vi "Servo MSMT Set Servo Type in Measurement Name.vi"(8 "error in (no error)":errorcluster, 11 "Servo to Power Out in":refnum<class "Servo to Power Out.lvclass">) -> (0 "error out":errorcluster, 3 "Servo to Power Out out":refnum<class "Servo to Power Out.lvclass">)   [LabVIEW 2018, in "Servo to Power Out.lvlib" / "Servo to Power Out.lvclass"]
uses:
  Servo to Power Out.lvclass
  C:/Sequence Automation/Plugins/Measurement Interface.lvlibp/Measurement Interface.lvclass
  Plugins/Measurement Interface.lvlibp/Private Methods/Measurement Name/Read Measurement Name.vi
  Plugins/Measurement Interface.lvlibp/Private Methods/Measurement Name/Write Measurement Name.vi
  Plugins/Measurements/Servo MSMT.lvlibp/Servo MSMT.lvclass
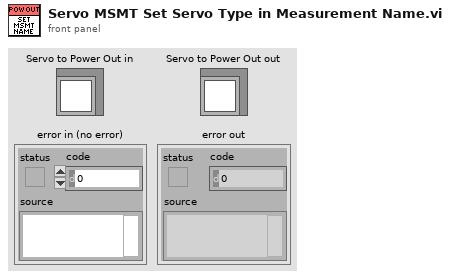
[diagram p1: front panel]
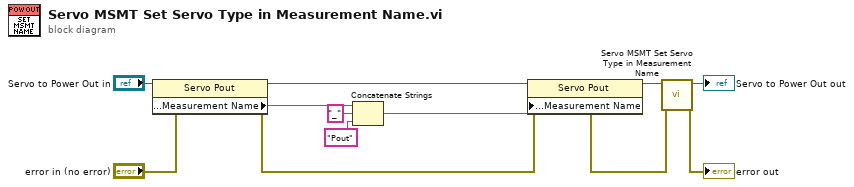
[diagram p0: block diagram]
diagram:
  n1 = property class="Servo Pout"(reference="Servo to Power Out in", error in="error in (no error)") -> (reference out=w6:refnum<class "Servo to Power Out.lvclass">, error out=w9:errorcluster, "Public Methods:Measurement Name"=w4:string)
  n2 = Concatenate Strings(w4, "_" ("string"), "Pout" ("string")) -> (w3:string)
  n3 = property class="Servo Pout"(reference=w6, error in=w9, "Public Methods:Measurement Name"=w3) -> (reference out=w5:refnum<class "Servo to Power Out.lvclass">, error out=w7:errorcluster)
  n4 = call-parent "Servo MSMT Set Servo Type in Measurement Name.vi"("error in (no error)"=w7, "Servo MSMT in"=w5) -> ("error out"=→"error out":errorcluster, "Servo MSMT out"=→"Servo to Power Out out":refnum<class "Servo to Power Out.lvclass">)  [unwired: 8 in]
